vi "Read Label.vi"(8 "error in (no error)":errorcluster, 11 "Message":refnum<class "ErrorMessage.lvclass">) -> (0 "error out":errorcluster, 2 "Label":string, 3 "Message":refnum<class "ErrorMessage.lvclass">)   [LabVIEW 2011, in "Messenging.lvlib" / "ErrorMessage.lvclass"]
uses:
  ErrorMessage.lvclass
  TextVarientMessage/MSG.lvclass
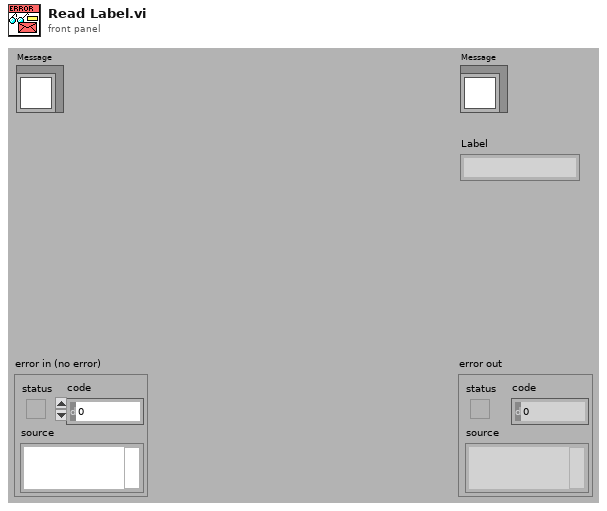
[diagram p1: front panel]
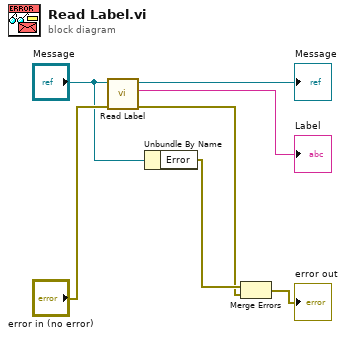
[diagram p0: block diagram]
diagram:
  n1 = call-parent "Read Label.vi"("error in (no error)"="error in (no error)", "Message"="Message") -> ("error out"=w1:errorcluster, "Label"=→"Label":string, "Message"=→"Message":refnum<class "ErrorMessage.lvclass">)  [unwired: 7 out]
  n2 = Unbundle By Name("Message") -> ("Error"=w2:errorcluster)
  n3 = Merge Errors(w2, w1) -> (→"error out":errorcluster)
